vi "DatabaseAPI-Update.vi"(0 "Database-API in":refnum<class "Database-API.lvclass">, 1 "data":variant, 2 "Where Statement":string, 5 "Update All":bool, 7 "Table":string, 9 "Column Number":i32, 11 "error in (no error)":errorcluster) -> (4 "Database-API out":refnum<class "Database-API.lvclass">, 15 "error out":errorcluster)   [LabVIEW 2014, in "Database-API.lvclass"]
uses:
  Database-API.lvclass
  Database-API.lvclass/Database-API.ctl
  <vilib>/addons/database/NI_Database_API.lvlib
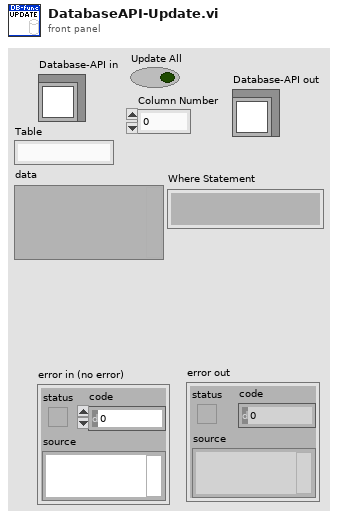
[diagram p1: front panel]
types:
  T1 = typedef "NI_Database_API.lvlib/Conn ObjectReference.ctl" = refnum<k1>
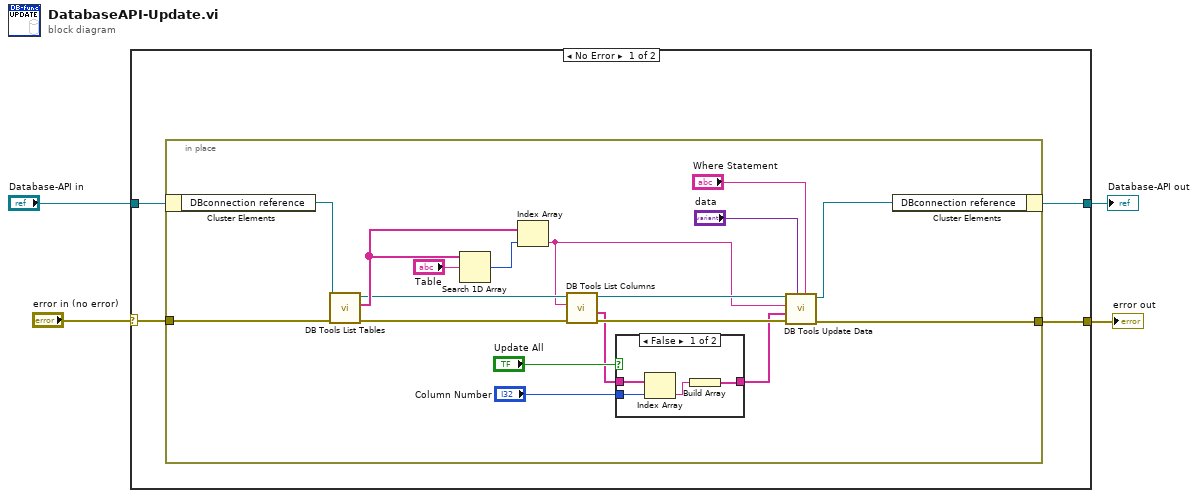
[diagram p0: block diagram]
diagram:
  n1 = case shown="No Error" "error in (no error)" {
    selector: "error in (no error)" -> [w6 w33]
    tunnel: [w5 w33] -> w3
    tunnel: [w7 w32] -> w1
    tunnel: "Database-API in" -> [w8 w32]
    frame No Error {
      n2 = in-place {
        in-place-border: w6 -> [w11]
        in-place-border: [w10] -> w5
        n3 = in-place-cluster #1(w8) -> ("DBconnection reference"=w26:T1)
        n4 = call <vilib>:"DB Tools List Tables.vi"("error in (no error)"=w11, "connection reference"=w26) -> ("error out"=w22:errorcluster, "tables"=w25:string[], "connection reference out"=w21:T1)  [unwired: 3 in]
        n5 = Search 1D Array(1D array=w25, element="Table") -> (index of element=w23:i32)  [unwired: 1 in]
        n6 = Index Array(array=w25, index=w23) -> (element=w15:string)
        n7 = call <vilib>:"DB Tools List Columns.vi"("error in (no error)"=w22, "table"=w15, "connection reference"=w21) -> ("error out"=w20:errorcluster, "columns"=w17:string[], "connection reference out"=w19:T1)  [unwired: 1 in, 1 out]
        n8 = case shown="False" "Update All" {
          tunnel: w17 -> [w30 w31]
          tunnel: [w27 w31] -> w16
          tunnel: "Column Number" -> [w29 _]
          frame False {
            n9 = Index Array(array=w30, index=w29) -> (element=w28:string)
            n10 = Build Array(w28) -> (w27:string[])
          }
          frame True {
          }
        }
        n11 = call <vilib>:"DB Tools Update Data.vi"("condition"="Where Statement", "data"="data", "error in (no error)"=w20, "columns"=w16, "table"=w15, "connection reference"=w19) -> ("error out"=w10:errorcluster, "connection reference out"=w12:T1)  [unwired: 4 in]
        n12 = in-place-cluster #1("DBconnection reference"=w12) -> (w7:refnum<class "Database-API.lvclass">)
      }
    }
    frame Error {
    }
  }
  "error out" <- w3
  "Database-API out" <- w1
